vi "Example_Robot_Simulation.vi"() -> ()   [LabVIEW 2019]
panel:
  in  "ControlR (-1 to 1)":dbl
  in  "ControlL (-1 to 1)":dbl min=-1.0 max=1.0 step=0.01
  out "SonarDistance":dbl
  in  "ServoAngle":dbl
  in  "IP Address":string="192.168.1.1"
  in  "Mode Select":T1(ring)=enum."Robot Simulation"
  out "Velocity Right":dbl
  out "Velocity Left":dbl
  in  "dt (ms)":u32=10
  in  "stop":bool
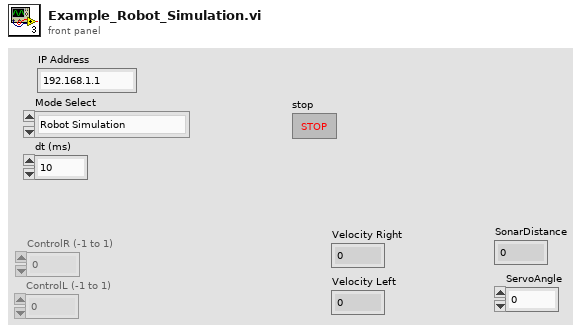
[diagram p1: front panel]
types:
  T1 = enum16{"Robot DC Motor Sim", "Robot Simulation", "Real Robot"}
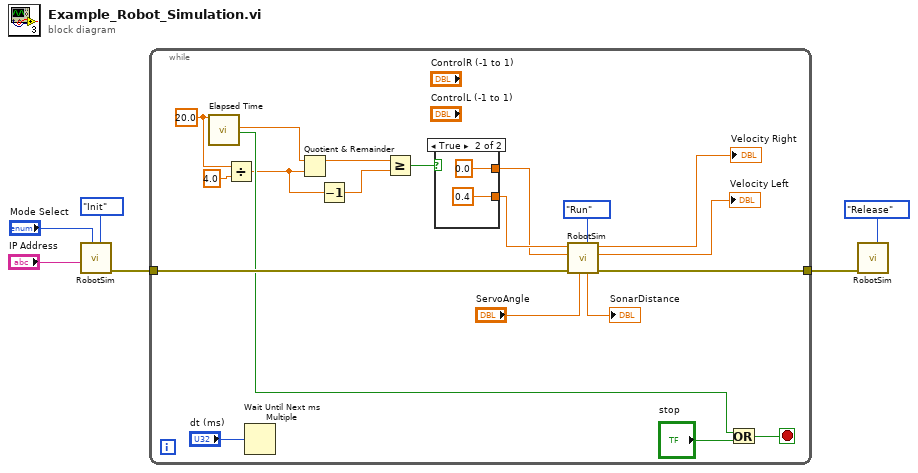
[diagram p0: block diagram]
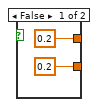
[diagram p2: hidden frame]
diagram:
  n1 = call "RobotSim.vi"("Action"=enum16{"Init", "Run", "Release"}."Init", "Mode Select"="Mode Select", "IP Address"="IP Address") -> ("error out"=w5:errorcluster)  [unwired: 4 in, 4 out]
  n2 = while {
    tunnel: w5 -> [w25]
    tunnel: [w23] -> w4
    stop <- w16 stop-if-true
    w15 = 20.0 ("Time Target (s)")
    n3 = call "Elapsed Time"("Time Target (s)"=w15) -> ("Elapsed Time (s)"=w14:dbl, "Time has Elapsed"=w13:bool)  [unwired: 11 in, 6 out]
    n4 = Divide(x=w15, y=4.0) -> (x/y=w7:dbl)
    n5 = Wait Until Next ms Multiple(millisecond multiple="dt (ms)") -> ()  [unwired: 1 out]
    n6 = Quotient & Remainder(x=w14, y=w7) -> (x-y*floor(x/y)=w8:dbl)  [unwired: 1 out]
    n7 = Decrement(x=w7) -> (x-1=w9:dbl)
    n8 = Greater Or Equal?(x=w8, y=w9) -> (x >= y?=w11:bool)
    n9 = case shown="True" w11 {
      tunnel: [0.2 ("ControlR") 0.4 ("ControlR")] -> w18
      tunnel: [0.2 ("ControlR") 0.0 ("ControlR")] -> w17
      frame False {
      }
      frame True {
      }
    }
    n10 = call "RobotSim.vi"("Action"=enum16{"Init", "Run", "Release"}."Run", "ServoAngle"="ServoAngle", "error in (no error)"=w25, "ControlL"=w17, "ControlR"=w18) -> ("error out"=w23:errorcluster, "OmegaL"=→"Velocity Left":dbl, "OmegaR"=→"Velocity Right":dbl, "SonarDistance"=→"SonarDistance":dbl)  [unwired: 2 in, 1 out]
    n11 = Or(x=w13, y="stop") -> (x .or. y?=w16:bool)
  }
  n12 = call "RobotSim.vi"("Action"=enum16{"Init", "Run", "Release"}."Release", "error in (no error)"=w4) -> ()  [unwired: 5 in, 5 out]
